vi "Get Earth Connection.vi"(8 "error in (no error)":errorcluster, 11 "VISA resource name":refnum<visa-resource-name>) -> (0 "error out":errorcluster, 2 "Earth Connection":u16, 3 "VISA resource name out":refnum<visa-resource-name>)   [LabVIEW 2013, in "Fluke 5XXX Series Multicalibrators.lvlib"]
doc: "This VI returns whether or not the Calibrator front panel NORMAL LO terminal is tied to chassis (earth) ground.\n\nNote:\n\nThis VI is available only for instrument models 5500A and 5520A."
uses:
  Fluke 5XXX Series Multicalibrators.lvlib
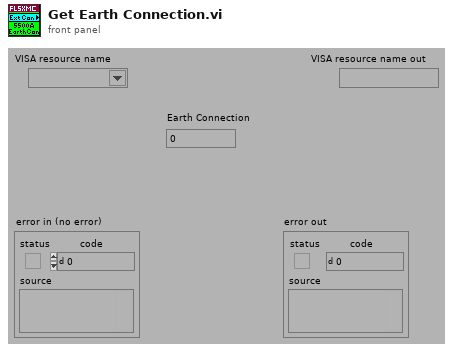
[diagram p1: front panel]
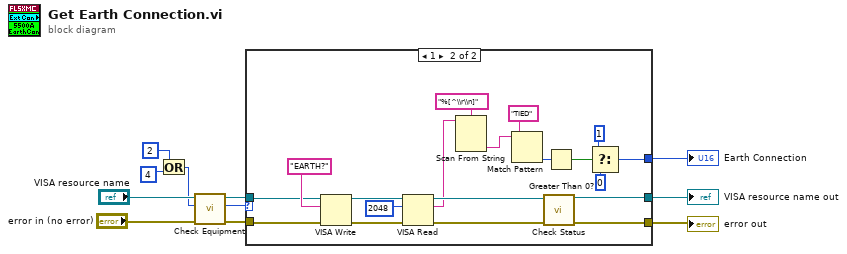
[diagram p0: block diagram]
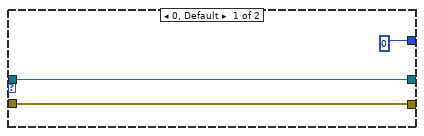
[diagram p2: hidden frame]
diagram:
  n1 = Or(x=2 ("Numeric"), y=4 ("Numeric")) -> (x .or. y?=w1:i32)
  n2 = call "Check Equipment.vi"("error in (no error)"="error in (no error)", "Bit Mask"=w1, "VISA resource name"="VISA resource name") -> ("error out"=w11:errorcluster, "Present?"=w10:u32, "VISA resource name out"=w9:refnum<visa-resource-name>)  [unwired: 6 in]
  n3 = case shown="1" w10 {
    tunnel: [w13 w27] -> w5
    tunnel: [w12 w24] -> w6
    tunnel: w11 -> [w13 w29]
    tunnel: w9 -> [w12 w28]
    tunnel: [u16 0 w15] -> w4
    frame 0, Default {
    }
    frame 1 {
      n4 = VISA Write(VISA resource name=w28, write buffer="EARTH?", error in (no error)=w29) -> (VISA resource name out=w32:refnum<visa-resource-name>, error out=w31:errorcluster)  [unwired: 1 out]
      n5 = VISA Read(VISA resource name=w32, byte count=u32 2048 ("byte count (0)"), error in (no error)=w31) -> (VISA resource name out=w25:refnum<visa-resource-name>, read buffer=w17:string, error out=w26:errorcluster)  [unwired: 1 out]
      n6 = Scan From String(format string="%[^\\r\\n]", input string=w17) -> (output 1=w16:string)  [unwired: 3 in, 3 out]
      n7 = Match Pattern(string=w16, regular expression="TIED") -> (offset past match=w21:i32)  [unwired: 1 in, 3 out]
      n8 = call "Check Status.vi"("VISA resource name"=w25, "error in (no error)"=w26) -> ("VISA resource name out"=w24:refnum<visa-resource-name>, "error out"=w27:errorcluster)  [unwired: 12 in]
      n9 = Greater Than 0?(x=w21) -> (x > 0?=w18:bool)
      n10 = Select(t=u16 1 ("f"), s=w18, f=u16 0) -> (s? t:f=w15:u16)
    }
  }
  "Earth Connection" <- w4
  "VISA resource name out" <- w6
  "error out" <- w5
